vi "MV_Set.vi"(8 "error in (no error)":errorcluster, 9 "Jog Mode":T1 items=["-666 steps/s"=-4, "-1700 steps/s"=-3, "-100 steps/s"=-2, "-5 steps/s"=-1, "No move"=0, "+5 steps/s"=1, "+100 steps/s"=2, "+1700 steps/s"=3, "+666 steps/s"=4], 10 "Axis Number":i32, 11 "Agilis in":T2) -> (0 "error out":errorcluster, 3 "Agilis out":T2)   [LabVIEW 2016, in "Drivers.lvlib" / "Agilis.lvlib"]
doc: "Starts a jog motion at a defined speed to the limit and stops automatically when the limit is activated."
uses:
  Agilis.lvlib
  AgilisCmdLib Refnum.ctl
  D:/Trace Grabber/Drivers/Agilis/AgilisCmdLib.dll
  AgilisCmdLib.dll
  Jog Mode.ctl
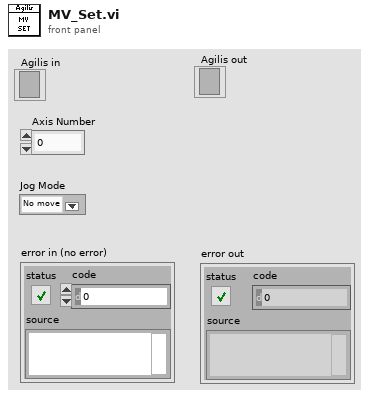
[diagram p1: front panel]
types:
  T1 = typedef "Drivers.lvlib/Agilis.lvlib/Jog Mode.ctl" = i32
  T2 = typedef "Drivers.lvlib/Agilis.lvlib/AgilisCmdLib Refnum.ctl" = refnum<k24>
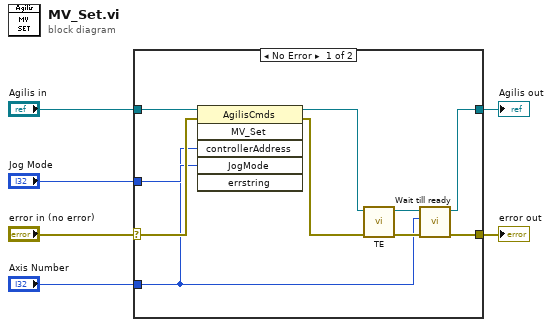
[diagram p0: block diagram]
diagram:
  n1 = case shown="No Error" "error in (no error)" {
    selector: "error in (no error)" -> [w15 w18]
    tunnel: "Agilis in" -> [w16 w17]
    tunnel: [w8 w17] -> w4
    tunnel: [w10 w18] -> w3
    tunnel: "Axis Number" -> [w7 _]
    tunnel: "Jog Mode" -> [w14 _]
    frame No Error {
      n2 = invoke class="AgilisCmds" method="MV_Set"(reference=w16, error in=w15, "controllerAddress"=w7, "JogMode"=w14) -> (reference out=w12:T2, error out=w13:errorcluster)  [unwired: 2 in, 4 out]
      n3 = call "TE.vi"("error in (no error)"=w13, "Agilis in"=w12) -> ("error out"=w11:errorcluster, "Agilis out"=w9:T2)  [unwired: 8 in]
      n4 = call "Wait till ready.vi"("error in (no error)"=w11, "Axis Number"=w7, ".NET Refnum in"=w9) -> ("error out"=w10:errorcluster, ".NET Refnum out"=w8:T2)  [unwired: 7 in]
    }
    frame Error {
    }
  }
  "Agilis out" <- w4
  "error out" <- w3
